vi "Limit.vi"(5 "XY_in":cluster{"压力":dbl[], "位移":dbl[]}(graph), 9 "边界配置":T1) -> (6 "XY_out":cluster{dbl[], dbl[]}[](graph), 10 "ok":bool)   [LabVIEW 2018]
panel:
  out "压力":dbl[](array[numeric])
  out "x > y?":bool
  out "a 4":dbl
  out "b 4":dbl
  out "b 3":dbl
  out "a 3":dbl
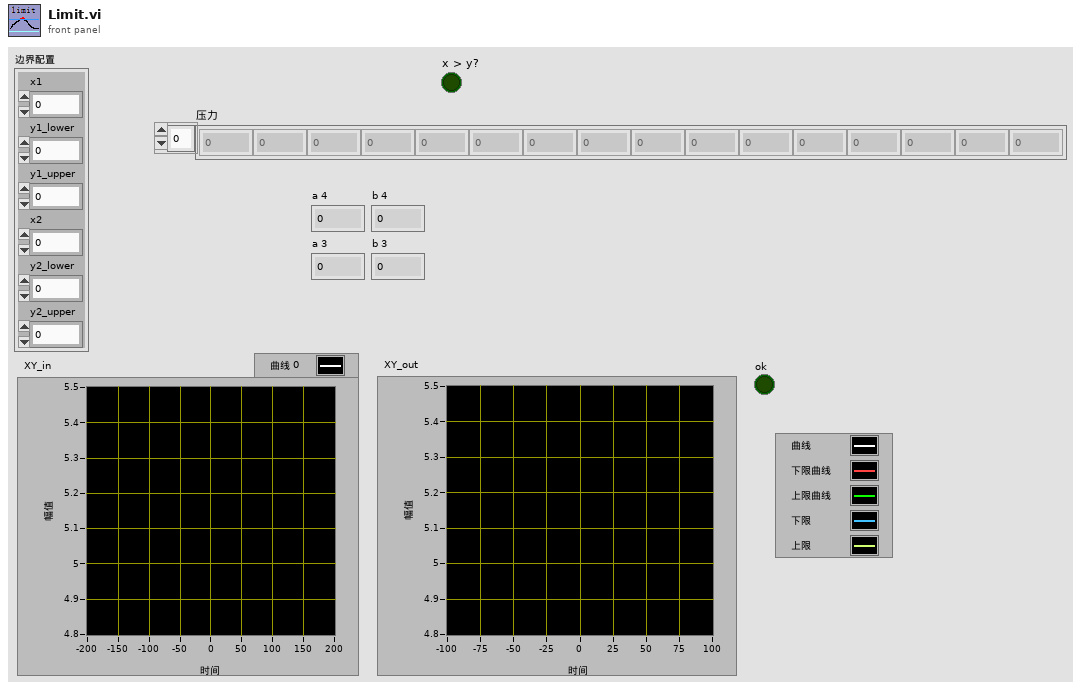
[diagram p1: front panel]
types:
  T1 = cluster{"x1":dbl, "y1_lower":dbl, "y1_upper":dbl, "x2":dbl, "y2_lower":dbl, "y2_upper":dbl}
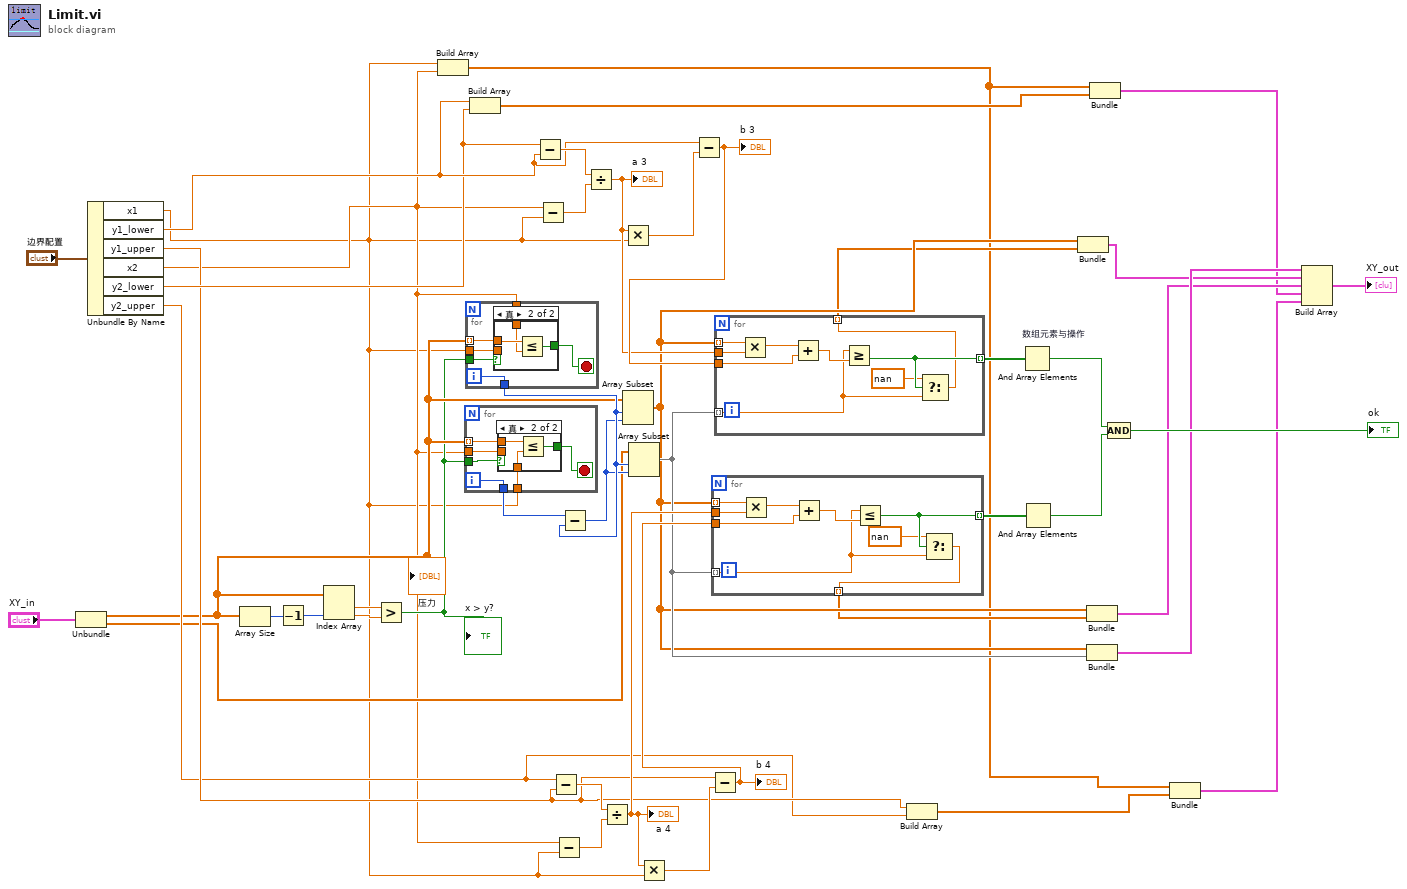
[diagram p0: block diagram]
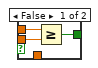
[diagram p2: hidden frame]
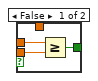
[diagram p3: hidden frame]
diagram:
  n1 = Unbundle("XY_in") -> ("压力"=w7:dbl[], "位移"=w9:dbl[])
  "压力" <- w7
  n2 = Unbundle By Name("边界配置") -> ("x1"=w1:dbl, "y1_lower"=w14:dbl, "y1_upper"=w12:dbl, "x2"=w2:dbl, "y2_lower"=w13:dbl, "y2_upper"=w11:dbl)
  n3 = Array Size(array=w7) -> (size(s)=w8:i32)
  n4 = Decrement(x=w8) -> (x-1=w6:i32)
  n5 = Index Array(array=w7, index #2=w6) -> (element #1=w5:dbl, element #2=w4:dbl)  [unwired: 1 in]
  n6 = Greater?(x=w5, y=w4) -> (0:w3:bool)
  "x > y?" <- w3
  n7 = Build Array(w1, w2) -> (w17:dbl[])
  n8 = for {
    tunnel: w7 -> [w52] mode=indexing
    tunnel: [w51] -> w31
    tunnel: w2 -> [w49]
    tunnel: w3 -> [w48]
    tunnel: w1 -> [w47]
    i -> [w51]
    stop <- w50 stop-if-true
    n9 = case shown="真" w48 {
      tunnel: w52 -> [w55 w58]
      tunnel: [w54 w57] -> w50
      tunnel: w49 -> [w53 _]
      tunnel: w47 -> [_ w56]
      frame False {
        n10 = Greater Or Equal?(x=w55, y=w53) -> (x >= y?=w54:bool)
      }
      frame True {
        n11 = Less Or Equal?(x=w58, y=w56) -> (x <= y?=w57:bool)
      }
    }
  }
  n12 = for {
    tunnel: w7 -> [w64] mode=indexing
    tunnel: [w63] -> w29
    tunnel: w3 -> [w61]
    tunnel: w1 -> [w60]
    tunnel: w2 -> [w59]
    i -> [w63]
    stop <- w62 stop-if-true
    n13 = case shown="真" w61 {
      tunnel: w64 -> [w67 w70]
      tunnel: [w66 w69] -> w62
      tunnel: w60 -> [w65 _]
      tunnel: w59 -> [_ w68]
      frame False {
        n14 = Greater Or Equal?(x=w67, y=w65) -> (x >= y?=w66:bool)
      }
      frame True {
        n15 = Less Or Equal?(x=w70, y=w68) -> (x <= y?=w69:bool)
      }
    }
  }
  n16 = Build Array(w14, w13) -> (w23:dbl[])
  n17 = Subtract(x=w13, y=w14) -> (x-y=w41:dbl)
  n18 = Subtract(x=w2, y=w1) -> (x-y=w40:dbl)
  n19 = Subtract(x=w11, y=w12) -> (x-y=w34:dbl)
  n20 = Subtract(x=w2, y=w1) -> (x-y=w35:dbl)
  n21 = Subtract(x=w31, y=w29) -> (x-y=w28:i32)
  n22 = Divide(x=w41, y=w40) -> (x/y=w37:dbl)
  "a 3" <- w37
  n23 = Divide(x=w34, y=w35) -> (x/y=w33:dbl)
  "a 4" <- w33
  n24 = Multiply(x=w37, y=w1) -> (x*y=w39:dbl)
  n25 = Array Subset(array=w7, index=w29, length=w28) -> (w26:dbl[])
  n26 = Array Subset(array=w9, index=w29, length=w28) -> (w27:dbl[])
  n27 = Multiply(x=w33, y=w1) -> (x*y=w36:dbl)
  n28 = Subtract(x=w14, y=w39) -> (x-y=w38:dbl)
  "b 3" <- w38
  n29 = Subtract(x=w12, y=w36) -> (x-y=w32:dbl)
  "b 4" <- w32
  n30 = for {
    tunnel: w26 -> [w79] mode=indexing
    tunnel: w27 -> [w71] mode=indexing
    tunnel: [w75] -> w45 mode=indexing
    tunnel: w33 -> [w77]
    tunnel: w32 -> [w76]
    tunnel: [w74] -> w24 mode=indexing
    n31 = Multiply(x=w79, y=w77) -> (x*y=w78:dbl)
    n32 = Add(x=w78, y=w76) -> (x+y=w73:dbl)
    n33 = Less Or Equal?(x=w71, y=w73) -> (x <= y?=w75:bool)
    n34 = Select(t=nan, s=w75, f=w71) -> (s? t:f=w74:dbl)
  }
  n35 = for {
    tunnel: w26 -> [w88] mode=indexing
    tunnel: w27 -> [w80] mode=indexing
    tunnel: [w84] -> w46 mode=indexing
    tunnel: w37 -> [w86]
    tunnel: w38 -> [w85]
    tunnel: [w83] -> w25 mode=indexing
    n36 = Multiply(x=w88, y=w86) -> (x*y=w87:dbl)
    n37 = Add(x=w87, y=w85) -> (x+y=w82:dbl)
    n38 = Greater Or Equal?(x=w80, y=w82) -> (x >= y?=w84:bool)
    n39 = Select(t=nan, s=w84, f=w80) -> (s? t:f=w83:dbl)
  }
  n40 = Build Array(w12, w11) -> (w18:dbl[])
  n41 = And Array Elements "数组元素与操作"(Boolean array=w46) -> (logical AND=w44:bool)
  n42 = And Array Elements(Boolean array=w45) -> (logical AND=w43:bool)
  n43 = Bundle(w26, w25) -> (w21:cluster{dbl[], dbl[]})  [unwired: 1 in]
  n44 = Bundle(w26, w24) -> (w20:cluster{dbl[], dbl[]})  [unwired: 1 in]
  n45 = Bundle(w26, w27) -> (w22:cluster{dbl[], dbl[]})  [unwired: 1 in]
  n46 = Bundle(w17, w23) -> (w19:cluster{dbl[], dbl[]})  [unwired: 1 in]
  n47 = Compound Arithmetic op=AND(w44, w43) -> (→"ok":bool)
  n48 = Bundle(w17, w18) -> (w16:cluster{dbl[], dbl[]})  [unwired: 1 in]
  n49 = Build Array(w22, w21, w20, w19, w16) -> (→"XY_out":cluster{dbl[], dbl[]}[])
